vi "Expand Type Def.vi"(8 "error in (no error)":errorcluster, 9 "Number of SPI Buses":i32, 10 "Device Channels":i32[](array[numeric]), 11 "Curent Bus Path":path) -> (0 "error out":errorcluster)   [LabVIEW 2014, in "Initialization and IO Node Scripting.lvlib"]
uses:
  Initialization and IO Node Scripting.lvlib
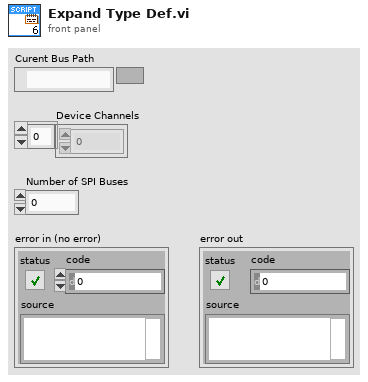
[diagram p1: front panel]
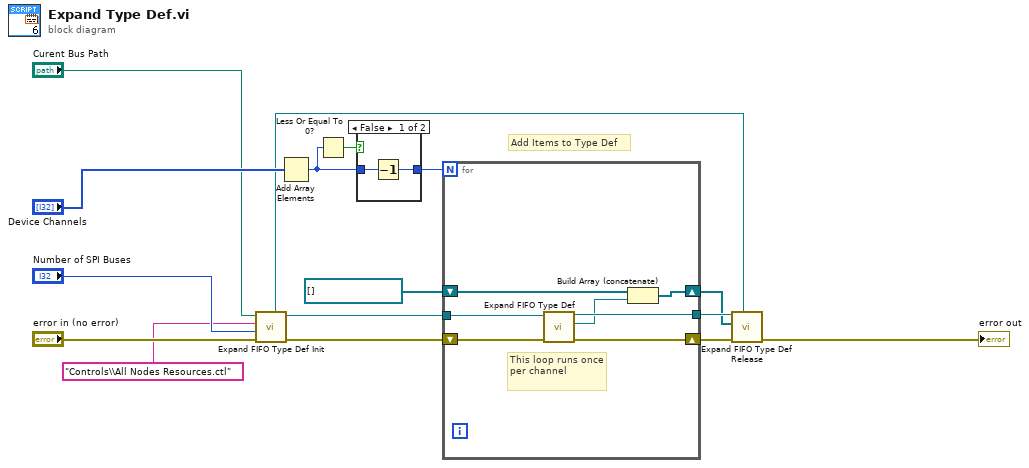
[diagram p0: block diagram]
diagram:
  # "Add Items to Type Def"
  n1 = call "Expand FIFO Type Def Init.vi"("error in (no error)"="error in (no error)", "Current Bus Number"="Number of SPI Buses", "Path to All Nodes Resources"="Controls\\All Nodes Resources.ctl", "Destination Path"="Curent Bus Path") -> ("error out"=w5:errorcluster, "Cluster out"=w6:refnum<vi>, "Control Refnum"=w11:refnum<vi>)  [unwired: 5 in]
  n2 = Add Array Elements(numeric array="Device Channels") -> (sum=w15:i32)
  n3 = Less Or Equal To 0?(x=w15) -> (x <= 0?=w13:bool)
  n4 = case shown="False" w13 {
    tunnel: w15 -> [w18 w19]
    tunnel: [w17 w19] -> w12
    frame False {
      n5 = Decrement(x=w18) -> (x-1=w17:i32)
    }
    frame True {
    }
  }
  n6 = for {
    N: w12 -> [_]
    shift-right: [w26] -> w4
    shift-left: w5 -> [w25]
    tunnel: w6 -> [w24]
    tunnel: [w23] -> w3
    shift-right: [w21] -> w2
    shift-left: refnum<vi>[] [] -> [w20]
    # "This loop runs once per channel"
    n7 = call "Expand FIFO Type Def.vi"("error in (no error)"=w25, "Cluster in"=w24) -> ("error out"=w26:errorcluster, "Clsuter Item"=w22:refnum<vi>, "Cluster out"=w23:refnum<vi>)  [unwired: 7 in]
    n8 = Build Array (concatenate)(w20, w22) -> (w21:refnum<vi>[])
  }
  n9 = call "Expand FIFO Type Def Release.vi"("Control Refnum"=w11, "error in (no error)"=w4, "Array"=w2, "Cluster in"=w3) -> ("error out"=→"error out":errorcluster)  [unwired: 7 in]
